vi "setColourRampScale.vi"(6 "scaleClipPercentile":dbl=1.0 format="%#_13g", 7 "Centre Value":T1(ring), 9 "comaparativeData":dbl[](array[numeric]), 11 "baselineData":dbl[](array[numeric])) -> (2 "colourRampVals":cluster{"value":dbl, "colour":u32}[](array[cluster]), 4 "whitePoint":dbl format="%0.2f")   [LabVIEW 2022 SP3]
uses:
  <vilib>/gmath/statdist.llb/st_Percentiles (scalar).vi
  <vilib>/Analysis/NI_AALBase.lvlib
  <vilib>/gmath/NI_Gmath.lvlib
panel:
  in  "median":cluster{"value":dbl, "colour":u32}={"value"=20.0, "colour"=16448250}
  in  "min":cluster{"value":dbl, "colour":u32}={"value"=10.0, "colour"=1015806}
  in  "max":cluster{"value":dbl, "colour":u32}={"value"=30.0, "colour"=16711680}
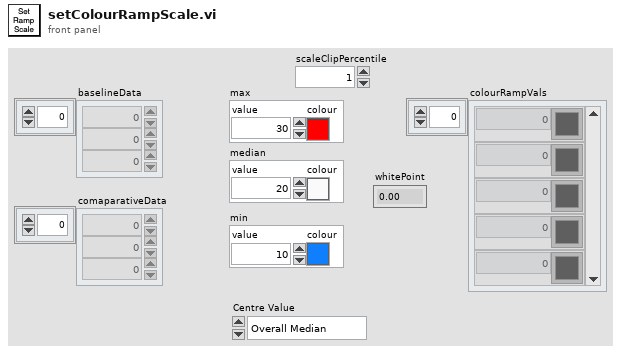
[diagram p1: front panel]
types:
  T1 = enum16{"Overall Median", "Baseline Median", "Zero"}
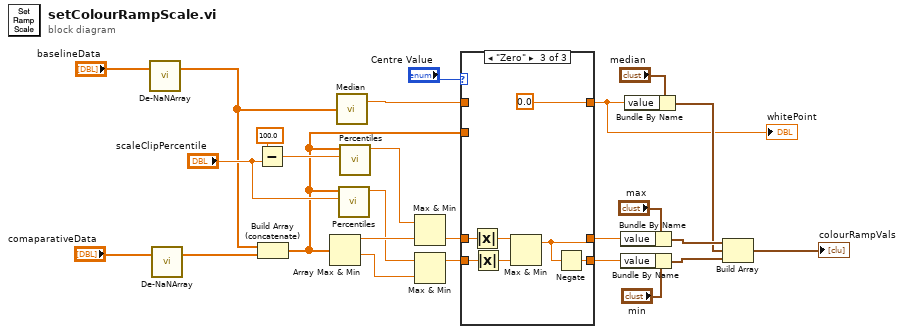
[diagram p0: block diagram]
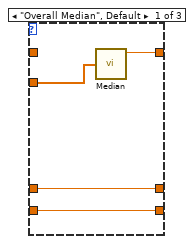
[diagram p2: hidden frame]
diagram:
  n1 = call "De-NaNArray.vi"("ArrayIn"="baselineData") -> ("de-NaN-dArrayOut"=w4:dbl[])  [unwired: 1 in, 1 out]
  n2 = call "De-NaNArray.vi"("ArrayIn"="comaparativeData") -> ("de-NaN-dArrayOut"=w2:dbl[])  [unwired: 1 in, 1 out]
  n3 = Subtract(x=100.0, y="scaleClipPercentile") -> (x-y=w18:dbl)
  n4 = Build Array (concatenate)(w4, w2) -> (w6:dbl[])
  n5 = Array Max & Min(array=w6) -> (max value=w15:dbl, min value=w14:dbl)  [unwired: 2 out]
  n6 = call <vilib>:"Median.vi"("X"=w4) -> ("median"=w10:dbl)  [unwired: 1 out]
  n7 = call-poly <vilib>:"Percentiles.vi"("p"="scaleClipPercentile", "x array"=w6) -> ("percentile"=w13:dbl)  [unwired: 8 in, 1 out]
  n8 = call-poly <vilib>:"Percentiles.vi"("p"=w18, "x array"=w6) -> ("percentile"=w16:dbl)  [unwired: 8 in, 1 out]
  n9 = Max & Min(x=w16, y=w15) -> (min(x,y)=w12:dbl)  [unwired: 1 out]
  n10 = Max & Min(x=w13, y=w14) -> (max(x,y)=w11:dbl)  [unwired: 1 out]
  n11 = case shown="\"Zero\"" "Centre Value" {
    tunnel: w12 -> [w30 w32 w40]
    tunnel: w11 -> [w29 w31 w39]
    tunnel: [w27 w33 0.0] -> w5
    tunnel: w10 -> [_ w33 _]
    tunnel: [w30 w32 w37] -> w9
    tunnel: [w29 w31 w36] -> w8
    tunnel: w6 -> [w28 _ _]
    frame "Overall Median", Default {
      n12 = call <vilib>:"Median.vi"("X"=w28) -> ("median"=w27:dbl)  [unwired: 1 out]
    }
    frame "Baseline Median" {
    }
    frame "Zero" {
      n13 = Absolute Value(x=w40) -> (abs(x)=w35:dbl)
      n14 = Absolute Value(x=w39) -> (abs(x)=w34:dbl)
      n15 = Max & Min(x=w35, y=w34) -> (max(x,y)=w37:dbl)  [unwired: 1 out]
      n16 = Negate(x=w37) -> (-x=w36:dbl)
    }
  }
  "whitePoint" <- w5
  n17 = Bundle By Name(cluster="max", "value"=w9) -> (w24:cluster{"value":dbl, "colour":u32})
  n18 = Bundle By Name(cluster="min", "value"=w8) -> (w21:cluster{"value":dbl, "colour":u32})
  n19 = Bundle By Name(cluster="median", "value"=w5) -> (w20:cluster{"value":dbl, "colour":u32})
  n20 = Build Array(w24, w20, w21) -> (→"colourRampVals":cluster{"value":dbl, "colour":u32}[])
